vi "Sandbox.vi"() -> ()   [LabVIEW 2016]
uses:
  <vilib>/NI Veristand/VeriStand Data/Library/VeriStand Data.lvlib
panel:
  out "Cast U64 Pointer":u64 format="%016x"
  out "Converted U64 Pointer":u64 format="%016x"
  out "Cast Double Pointer":dbl
  out "Converted Double Pointer":dbl
  out "Original Pointer":u64 format="%016x"
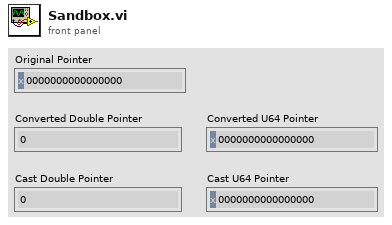
[diagram p1: front panel]
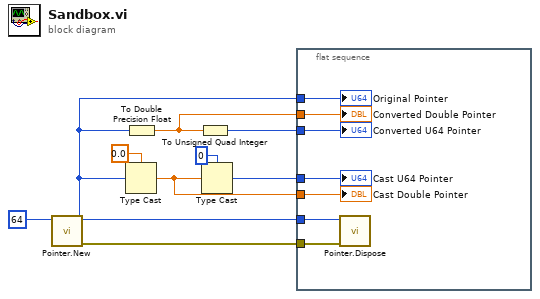
[diagram p0: block diagram]
diagram:
  n1 = call <vilib>:"Pointer.New.vi"("size in bytes"=64) -> ("error out"=w9:errorcluster, "pointer"=w1:u64)  [unwired: 9 in]
  n2 = Type Cast(type=0.0, x=w1) -> (*(type *) &x=w5:dbl)
  n3 = To Double Precision Float(number=w1) -> (double precision float=w7:dbl)
  n4 = To Unsigned Quad Integer(1:w7) -> (0:w6:u64)
  n5 = Type Cast(type=u64 0, x=w5) -> (*(type *) &x=w2:u64)
  n6 = flat-sequence {
    tunnel: w9 -> [w16]
    tunnel: w7 -> [w15]
    tunnel: w6 -> [w11]
    tunnel: w1 -> [w14]
    tunnel: w5 -> [w13]
    tunnel: w2 -> [w10]
    tunnel: w1 -> [w12]
    frame #0 {
      n7 = call <vilib>:"Pointer.Dispose.vi"("error in (no error)"=w16, "pointer"=w14) -> ()  [unwired: 8 in, 2 out]
      "Original Pointer" <- w12
      "Converted Double Pointer" <- w15
      "Cast Double Pointer" <- w13
      "Converted U64 Pointer" <- w11
      "Cast U64 Pointer" <- w10
    }
  }
